vi "CheckSingleCmdTest.vi"() -> ()   [LabVIEW 2014]
panel:
  in  "CMD array":u32[](array[numeric]) format="%032b"
  out "outbit_in":bool
  out "outbit_out":bool
  out "curScan":i32
  out "curStep":i32
  in  "stop":bool
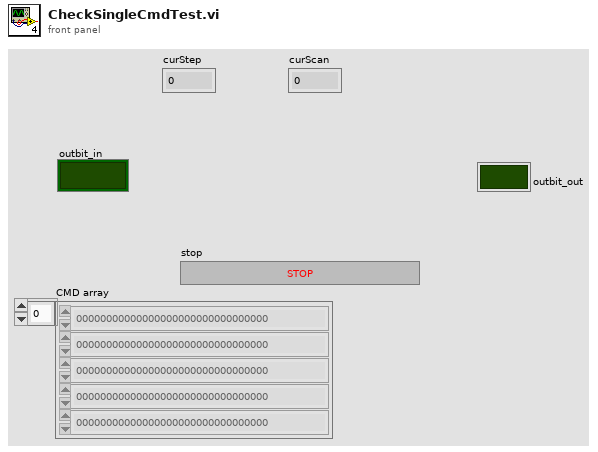
[diagram p1: front panel]
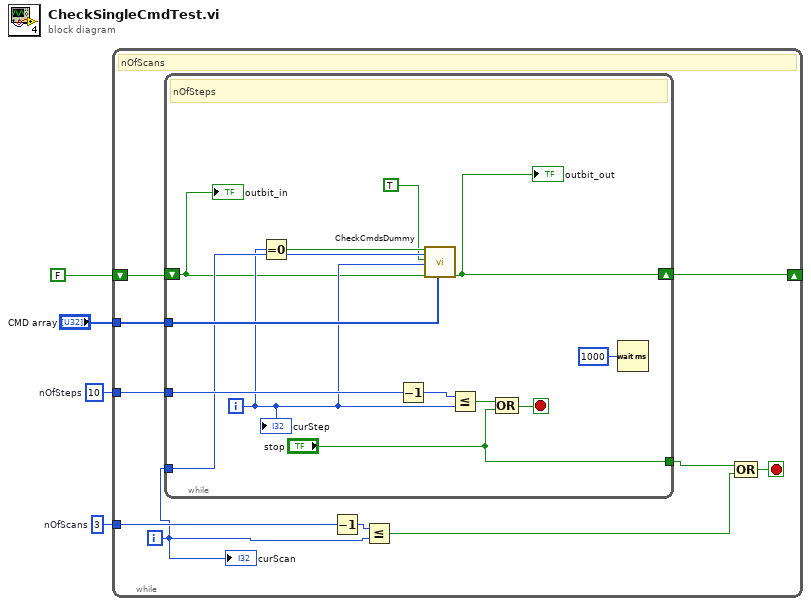
[diagram p0: block diagram]
diagram:
  w3 = 3  # nOfScans
  w4 = 10  # nOfSteps
  n1 = while {
    tunnel: w3 -> [w11]
    tunnel: w4 -> [w10]
    shift-right: [w6] -> _
    shift-left: FALSE ("outbit_out") -> [w8]
    tunnel: "CMD array" -> [w5]
    i -> [w7]
    stop <- w13 stop-if-true
    # "nOfScans"
    n2 = while {
      tunnel: w10 -> [w25]
      tunnel: ["stop"] -> w9
      shift-right: [w15] -> w6
      shift-left: w8 -> [w16]
      tunnel: w7 -> [w19]
      tunnel: w5 -> [w21]
      i -> [w17]
      stop <- w24 stop-if-true
      # "nOfSteps"
      n3 = Equal To 0?(x=w17) -> (x = 0?=w20:bool)
      n4 = Decrement(x=w25) -> (x-1=w27:i32)
      n5 = call "CheckCmdsDummy.vi"("scanChanged"=w20, "actScan"=w19, "stepChanged"=TRUE, "actStep"=w17, "outbit_iN"=w16, "CMD array"=w21) -> ("outbit_out"=w15:bool)  [unwired: 13 in]
      "outbit_out" <- w15
      n6 = Less Or Equal?(x=w27, y=w17) -> (x <= y?=w26:bool)
      n7 = Compound Arithmetic op=OR(w26, "stop") -> (w24:bool)
      n8 = Wait (ms)(milliseconds to wait=u32 1000) -> ()  [unwired: 1 out]
      "curStep" <- w17
      "outbit_in" <- w16
    }
    n9 = Decrement(x=w11) -> (x-1=w12:i32)
    n10 = Less Or Equal?(x=w12, y=w7) -> (x <= y?=w14:bool)
    n11 = Compound Arithmetic op=OR(w9, w14) -> (w13:bool)
    "curScan" <- w7
  }
